vi "Dispose VISA Lock Ref.vi"(8 "error in (no error)":errorcluster, 10 "release all (F)":bool, 11 "VISA session in":refnum<visa-resource-name>) -> (0 "error out":errorcluster, 3 "VISA session out":refnum<visa-resource-name>)   [LabVIEW 2021, in "MB_VISA_Lock.lvlib"]
doc: "Dispose of the VISA resource lock reference. The output VISA session will have an invalid reference stored in the User Data property. This VI should be called just before closing the VISA session.\n\nInput errors do not affect the behavior of this VI."
uses:
  <vilib>/Plasmionique/MB Master/MB_VISA_Lock/MB_VISA_Lock.lvlib
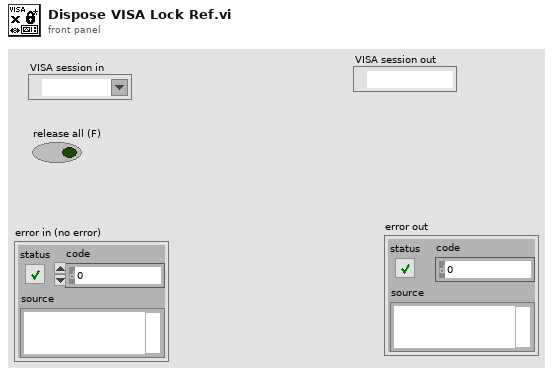
[diagram p1: front panel]
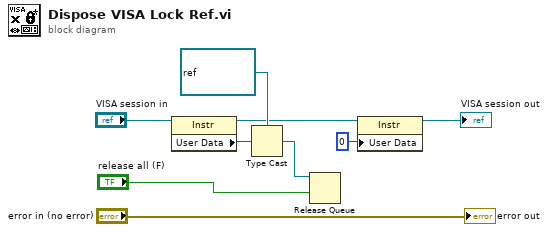
[diagram p0: block diagram]
diagram:
  n1 = property class="Instr"(reference="VISA session in") -> (reference out=w5:refnum<visa-resource-name>, "User Data"=w8:u32)  [unwired: 1 in, 1 out]
  n2 = Type Cast(type=refnum<queue> refnum ("lock ref out"), x=w8) -> (*(type *) &x=w6:refnum<queue>)
  n3 = Release Queue(queue=w6, force destroy? (F)="release all (F)") -> ()  [unwired: 1 in, 3 out]
  n4 = property class="Instr"(reference=w5, "User Data"=u32 0 ("General Settings:User Data")) -> (reference out=→"VISA session out":refnum<visa-resource-name>)  [unwired: 1 in, 1 out]
  "error out" <- "error in (no error)"
